vi "PH_Sixpack.Action Init or Close.vi"(0 "VI in":refnum<vi>, 5 "error in":errorcluster) -> (14 "VI out":refnum<vi>, 19 "error out":errorcluster)   [LabVIEW 2014, in "PH_Sixpack.lvlib"]
doc: "This VI is made to act on 6P hardware in a certain state. It is used in ProcPrdc."
uses:
  PH_Sixpack.lvlib
  PH_Sixpack.Status.ctl
  PH_Common/PH_Common.lvlib
  PH_Stepmotor_BaseClass/PH_Stepmotor_BaseClass.lvlib
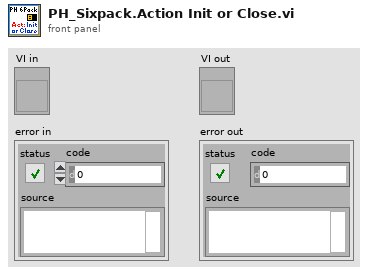
[diagram p1: front panel]
types:
  T1 = typedef "PH_Sixpack.lvlib/PH_Sixpack.Status.ctl" = enum32{"None", "Init", "Configure", "configured", "Close", "closed"}
  T2 = typedef "PH_Sixpack.lvlib/PH_Sixpack.i attribute.ctl" = cluster{"Information":cluster{"SixPack ID(0)":u16, "BaudRate(19200)":u16, "COM Port":enum32{"COM1", "COM2", "COM3", "COM4", "COM5", "COM6", "COM7", "COM8", "COM9"}, "HANDLE":i32}, "Serial Number":dbl, "Firmwareversion":dbl, "Axes":T3[], "Status":T1, "Axis to do a RefSearch":i32, "GUI Refs":cluster{"Information":refnum<vi>, "Serial Number":refnum<vi>, "Firmwareversion":refnum<vi>, "Status":refnum<vi>, "Axis to do a RefSearch":refnum<vi>, "Axes Configuration (Sixpack)":refnum<vi>, "Inputs":refnum<vi>, "PeriodicInterval [ms]":refnum<vi>}, "Constructor finished":bool, "Ignore Error":bool}
  T3 = typedef "PH_Sixpack.lvlib/PH_Sixpack.Axis Cluster.ctl" = cluster{"Config":T4, "To set?":cluster{"VmaxAmax":bool, "I max":bool, "VStartVminDivi":bool, "Ref Search Parameter":bool, "Stopswitch Limits":bool, "Axis Parameter":bool, "I Control":bool}}
  T4 = typedef "PH_Sixpack.lvlib/PH_Sixpack.Axis Configuration.ctl" = cluster{"VmaxAmax":T5, "I max (50%)":T6, "VStartVminDivi":T7, "Ref Search Parameter":T8, "Stopswitch Limits":T9, "Axis Parameter":T10, "I Control":T13}
  T5 = typedef "Sixpack - Driver.lvlib/VmaxAmax.ctl" = cluster{"VMax(511)":u16, "AMax(128)":u16}
  T6 = typedef "Sixpack - Driver.lvlib/PeakCurrent.ctl" = dbl
  T7 = typedef "Sixpack - Driver.lvlib/VStartVmin.ctl" = cluster{"VStart(5)":u16, "Vmin(4)":u16, "Div i (2)":enum8{"0", "1", "2", "3"}}
  T8 = typedef "Sixpack - Driver.lvlib/Ref Search Parameter.ctl" = cluster{"VRefMax(100)":u16, "DebouncingTime (22ms)":u8}
  T9 = typedef "Sixpack - Driver.lvlib/Stopswitch Limits.ctl" = cluster{"MinLeft(0)":u16, "MaxRight(1023)":u16}
  T10 = typedef "Sixpack - Driver.lvlib/Motor Parameter.ctl" = cluster{"Poslimit (6400)":u32, "P5 Bits":T11, "P6 Bits":T12}
  T11 = typedef "Sixpack - Driver.lvlib/MotorParameter_P5.ctl" = cluster{"MT_PI":bool, "MT_ROTARY":bool, "MT_AUTONULLCMD":bool, "MT_TESTNULL":bool, "MT_NULLLEFT":bool, "MT_NULLCENTRE":bool, "MT_STOPNULL":bool, "MT_FILTERSWITCH":bool}
  T12 = typedef "Sixpack - Driver.lvlib/MotorParameter_P6.ctl" = cluster{"MT_OPTIMIZEWAY":bool, "MT_FASTREF":bool, "MT_MECHREF":bool, "MT_DELAYTESTNULL":bool, "MT_STOPSOFT":bool, "MT_STOPNOREF":bool, "MT_NULLPOSITIVE":bool, "MUT_STOPFULSTEPS":bool}
  T13 = typedef "Sixpack - Driver.lvlib/Current Control.ctl" = cluster{"PowerDownDelay (500)":u16, "PowerDown (0%)":T14, "Standing (50%)":T14, "Running (75%)":T14, "Accelerating (100%)":T14}
  T14 = typedef "Sixpack - Driver.lvlib/Current.ctl" = enum8{"100%", "75%", "50%", "38%", "25%", "19%", "13%", "9%", "0%"}
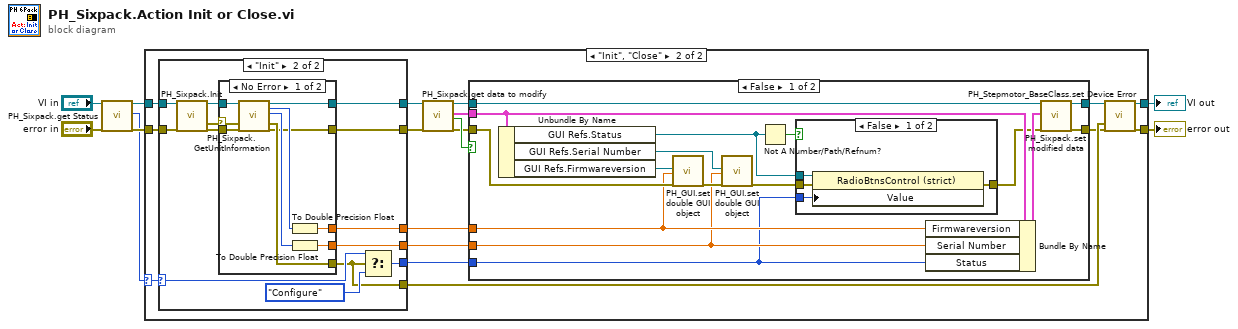
[diagram p0: block diagram]
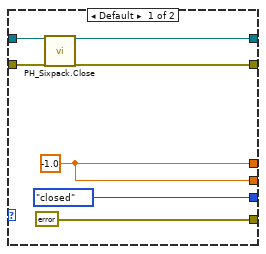
[diagram p3: hidden frame]
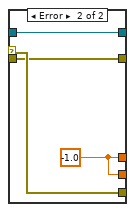
[diagram p4: hidden frame]
diagram:
  n1 = call "PH_Sixpack.get Status.vi"("VI in"="VI in", "error in (no error)"="error in") -> ("VI out"=w4:refnum<vi>, "Status"=w1:T1, "error out"=w2:errorcluster)  [unwired: 14 in, 1 out]
  n2 = case shown="\"Init\", \"Close\"" w1 {
    selector: w1 -> [_ w16]
    tunnel: w4 -> [w9 w26]
    tunnel: w2 -> [w8 w25]
    tunnel: [w8 w11] -> w6
    tunnel: [w9 w13] -> w7
    frame Default {
    }
    frame "Init", "Close" {
      n3 = case shown="\"Init\"" w16 {
        selector: w16 -> [_ w35]
        tunnel: w26 -> [w32 w44]
        tunnel: w25 -> [w31 w43]
        tunnel: [PH_Sixpack.Status."closed" ("Status") w42] -> w15
        tunnel: [w30 w36] -> w20
        tunnel: [w29 w37] -> w19
        tunnel: [w28 w39] -> w18
        tunnel: [w28 w38] -> w17
        tunnel: [errorcluster {"status"=FALSE, "code"=0, "source"=""} ("error IO") w34] -> w14
        frame Default {
          w28 = -1.0
          n4 = call "PH_Sixpack.Close.vi"("i ref in"=w32, "error in (no error)"=w31) -> ("i ref out"=w29:refnum<vi>, "error out"=w30:errorcluster)  [unwired: 16 in]
        }
        frame "Init" {
          n5 = call "PH_Sixpack.Init.vi"("i ref in"=w44, "error in"=w43) -> ("i ref out"=w45:refnum<vi>, "Device Error out"=w40:errorcluster, "error out"=w46:errorcluster)  [unwired: 15 in]
          n6 = case shown="No Error" w40 {
            selector: w40 -> [w49 w60]
            tunnel: w46 -> [w56 w59]
            tunnel: w45 -> [w55 w58]
            tunnel: [w52 w60] -> w34
            tunnel: [w51 w58] -> w37
            tunnel: [w50 w59] -> w36
            tunnel: [w48 w57] -> w39
            tunnel: [w47 w57] -> w38
            frame No Error {
              n7 = call "PH_Sixpack.GetUnitInformation.vi"("i ref in"=w55, "Device Error in"=w49, "error in (no error)"=w56) -> ("i ref out"=w51:refnum<vi>, "FirmawareVersion"=w53:u8, "Serial Number"=w54:u16, "Device Error out"=w52:errorcluster, "error out"=w50:errorcluster)  [unwired: 10 in, 2 out]
              n8 = To Double Precision Float(number=w53) -> (double precision float=w48:dbl)
              n9 = To Double Precision Float(number=w54) -> (double precision float=w47:dbl)
            }
            frame Error {
              w57 = -1.0
            }
          }
          n10 = Select(t=w35, s=w34, f=PH_Sixpack.Status."Configure" ("Status")) -> (s? t:f=w42:T1)
        }
      }
      n11 = call "PH_Sixpack.get data to modify.vi"("i ref in"=w19, "error in (no error)"=w20) -> ("i ref out"=w22:refnum<vi>, "i attribute"=w24:T2, "timed out"=w23:bool, "error out"=w21:errorcluster)  [unwired: 14 in]
      n12 = case shown="False" w23 {
        tunnel: w21 -> [w71 w82]
        tunnel: [w76 w82] -> w10
        tunnel: w22 -> [w75 w83]
        tunnel: [w74 w83] -> w12
        tunnel: w24 -> [w69 _]
        tunnel: w18 -> [w66 _]
        tunnel: w17 -> [w65 _]
        tunnel: w15 -> [w63 _]
        frame False {
          n13 = Unbundle By Name(w69) -> ("GUI Refs.Status"=w62:refnum<vi>, "GUI Refs.Serial Number"=w67:refnum<vi>, "GUI Refs.Firmwareversion"=w68:refnum<vi>)
          n14 = call "PH_GUI.set double GUI object.vi"("GUI object Ref"=w68, "value"=w66, "error in (no error)"=w71) -> ("error out"=w70:errorcluster)  [unwired: 16 in]
          n15 = call "PH_GUI.set double GUI object.vi"("GUI object Ref"=w67, "value"=w65, "error in (no error)"=w70) -> ("error out"=w72:errorcluster)  [unwired: 16 in]
          n16 = Not A Number/Path/Refnum?(number/path/refnum=w62) -> (NaN/Path/Refnum?=w61:bool)
          n17 = case shown="False" w61 {
            tunnel: w72 -> [w80 w81]
            tunnel: [w79 w81] -> w64
            tunnel: w62 -> [w78 _]
            tunnel: w63 -> [w77 _]
            frame False {
              n18 = property class="RadioBtnsControl (strict)"(reference=w78, error in=w80, "Value"=w77) -> (error out=w79:errorcluster)  [unwired: 1 out]
            }
            frame True {
            }
          }
          n19 = Bundle By Name(cluster=w69, "Firmwareversion"=w66, "Serial Number"=w65, "Status"=w63) -> (w73:T2)
          n20 = call "PH_Sixpack.set modified data.vi"("i ref in"=w75, "i attribute"=w73, "error in (no error)"=w64) -> ("i ref out"=w74:refnum<vi>, "error out"=w76:errorcluster)  [unwired: 15 in]
        }
        frame True {
        }
      }
      n21 = call "PH_Stepmotor_BaseClass.set Device Error.vi"("i ref in"=w12, "Device Error"=w14, "error in"=w10) -> ("i ref out"=w13:refnum<vi>, "error out"=w11:errorcluster)  [unwired: 15 in]
    }
  }
  "error out" <- w6
  "VI out" <- w7
